vi "BlkReadFrame.vi"(0 "引用句柄输入":refnum<file>, 1 "datatype":i32, 2 "DST":T1, 3 "FrameWidth":i32, 4 "SkipFrame":i32, 5 "FrameHeight":i32) -> (6 "Image out":T1(plugin-control))   [LabVIEW 2011]
uses:
  <vilib>/vision/Image Controls.llb/IMAQ Image.ctl
panel:
  in  "数值 4":u8
  in  "数值 3":u32
  in  "数值 2":i16
  in  "数值":sgl
  in  "错误输入":errorcluster
  out "错误输出":errorcluster
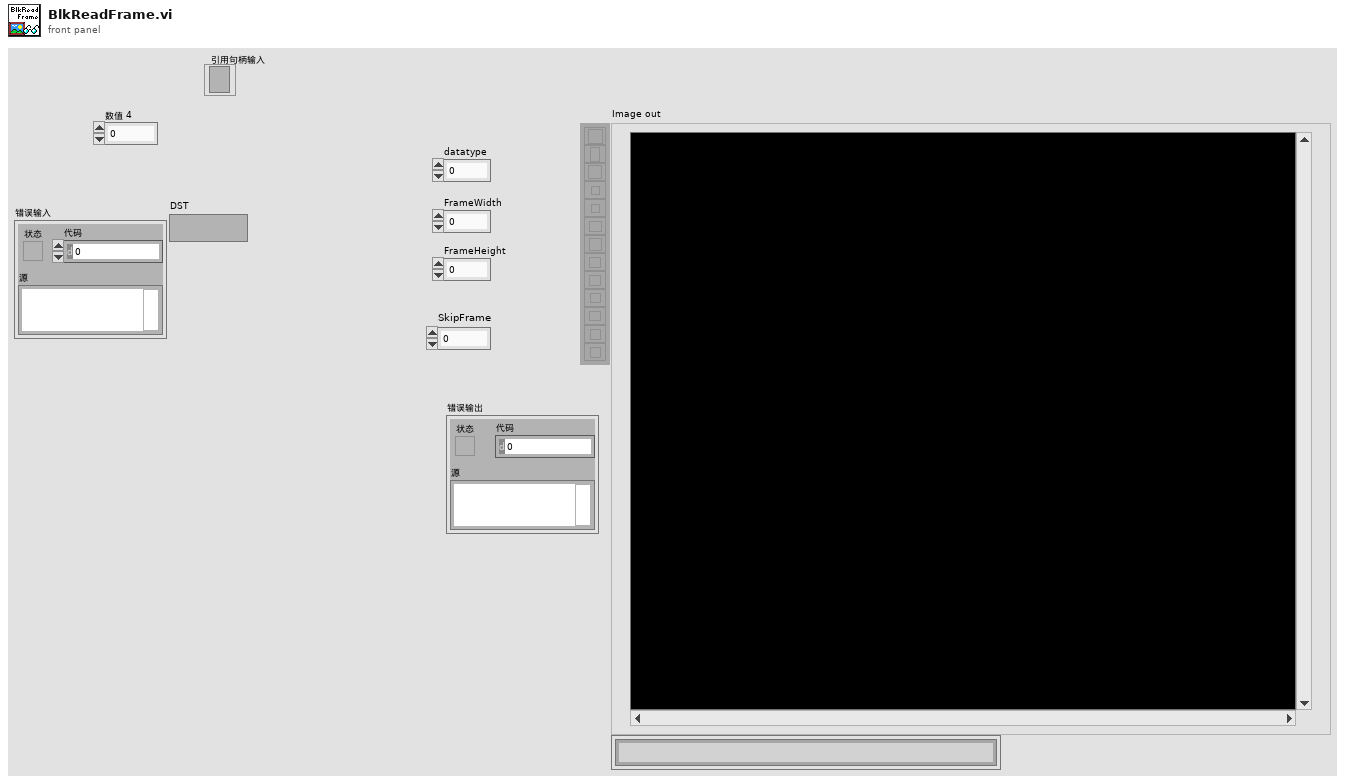
[diagram p1: front panel]
types:
  T1 = typedef "IMAQ Image.ctl" = refnum<image>
  T2 = enum16{"big-endian, network order", "native, host order", "little-endian"}
  T3 = typedef "Image Type" = u32
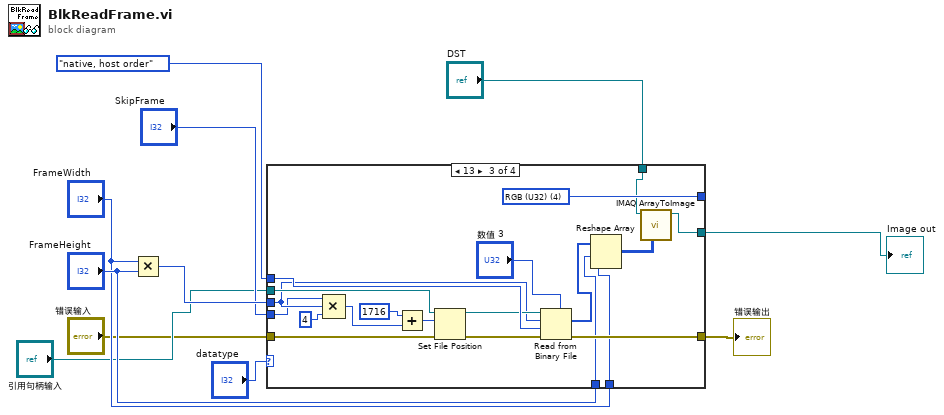
[diagram p0: block diagram]
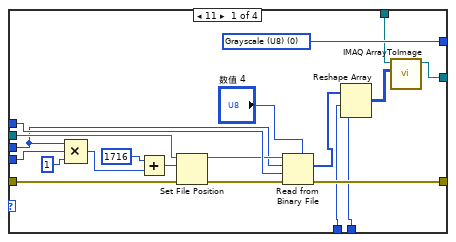
[diagram p2: hidden frame]
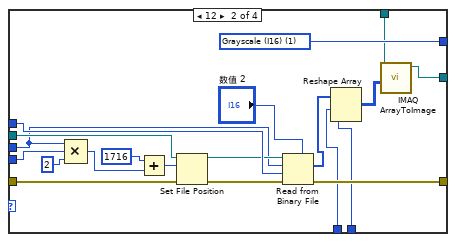
[diagram p3: hidden frame]
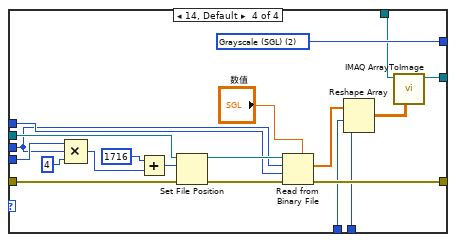
[diagram p4: hidden frame]
diagram:
  n1 = Multiply(x="FrameWidth", y="FrameHeight") -> (x*y=w8:i32)
  n2 = case shown="13" "datatype" {
    tunnel: [w31 w51 w71 w91] -> w11
    tunnel: T2."native, host order" ("字节顺序(0:big-endian, network order)") -> [w29 w49 w69 w80]
    tunnel: w8 -> [w18 w38 w61 w78]
    tunnel: [w28 w48 w68 w89] -> _
    tunnel: "错误输入" -> [w20 w40 w65 w82]
    tunnel: "引用句柄输入" -> [w21 w41 w64 w81]
    tunnel: "SkipFrame" -> [w19 w39 w58 w79]
    tunnel: "FrameHeight" -> [w15 w36 w55 w75]
    tunnel: "FrameWidth" -> [w14 w35 w54 w74]
    tunnel: "DST" -> [w12 w34 w53 w73]
    tunnel: [w17 w32 w52 w72] -> w3
    frame 11 {
      w28 = T3 0 items=["Grayscale (U8)", "Grayscale (I16)", "Grayscale (SGL)", "Complex (CSG)", "RGB (U32)", "HSL (U32)", "RGB (U64)", "Grayscale (U16)"] ("Image Type")
      n3 = Compound Arithmetic op=MULTIPLY(w18, w19, 1 ("y")) -> (w24:i32)
      n4 = Add(x=i64 1716 ("偏移量（字节）（0） 2"), y=w24) -> (x+y=w26:i64)
      n5 = Set File Position(offset (in bytes) (0)=w26, refnum=w21, error in=w20) -> (refnum out=w23:refnum<file>, error out=w22:errorcluster)  [unwired: 1 in]
      n6 = Read from Binary File(5:"数值 4", 8:w22, 9:w29, 10:w18, 11:w23) -> (0:w31:errorcluster, 2:w16:u8[])  [unwired: 1 in, 2 out]
      n7 = Reshape Array(w16, w15, w14) -> (w13:u8[][])
      n8 = call "IMAQ ArrayToImage"("Image Pixels (U8)"=w13, "Image"=w12) -> ("Image Out"=w17:T1)  [unwired: 8 in, 1 out]
    }
    frame 12 {
      w48 = T3 1 items=["Grayscale (U8)", "Grayscale (I16)", "Grayscale (SGL)", "Complex (CSG)", "RGB (U32)", "HSL (U32)", "RGB (U64)", "Grayscale (U16)"] ("Image Type")
      n9 = Compound Arithmetic op=MULTIPLY(w38, w39, 2 ("y")) -> (w44:i32)
      n10 = Add(x=i64 1716 ("偏移量（字节）（0） 2"), y=w44) -> (x+y=w46:i64)
      n11 = Set File Position(offset (in bytes) (0)=w46, refnum=w41, error in=w40) -> (refnum out=w43:refnum<file>, error out=w42:errorcluster)  [unwired: 1 in]
      n12 = Read from Binary File(5:"数值 2", 8:w42, 9:w49, 10:w38, 11:w43) -> (0:w51:errorcluster, 2:w37:i16[])  [unwired: 1 in, 2 out]
      n13 = Reshape Array(w37, w36, w35) -> (w33:i16[][])
      n14 = call "IMAQ ArrayToImage"("Image Pixels (I16)"=w33, "Image"=w34) -> ("Image Out"=w32:T1)  [unwired: 8 in, 1 out]
    }
    frame 13 {
      w68 = T3 4 items=["Grayscale (U8)", "Grayscale (I16)", "Grayscale (SGL)", "Complex (CSG)", "RGB (U32)", "HSL (U32)", "RGB (U64)", "Grayscale (U16)"] ("Image Type")
      n15 = Compound Arithmetic op=MULTIPLY(w58, w61, 4 ("y")) -> (w59:i32)
      n16 = Add(x=i64 1716 ("偏移量（字节）（0） 2"), y=w59) -> (x+y=w62:i64)
      n17 = Set File Position(offset (in bytes) (0)=w62, refnum=w64, error in=w65) -> (refnum out=w67:refnum<file>, error out=w66:errorcluster)  [unwired: 1 in]
      n18 = Read from Binary File(5:"数值 3", 8:w66, 9:w69, 10:w61, 11:w67) -> (0:w71:errorcluster, 2:w56:u32[])  [unwired: 1 in, 2 out]
      n19 = Reshape Array(w56, w55, w54) -> (w57:u32[][])
      n20 = call "IMAQ ArrayToImage"("Image Pixels (Float)"=w57, "Image"=w53) -> ("Image Out"=w52:T1)  [unwired: 8 in, 1 out]
    }
    frame 14, Default {
      w89 = T3 2 items=["Grayscale (U8)", "Grayscale (I16)", "Grayscale (SGL)", "Complex (CSG)", "RGB (U32)", "HSL (U32)", "RGB (U64)", "Grayscale (U16)"] ("Image Type")
      n21 = Compound Arithmetic op=MULTIPLY(w79, w78, 4 ("y")) -> (w85:i32)
      n22 = Add(x=i64 1716 ("偏移量（字节）（0） 2"), y=w85) -> (x+y=w87:i64)
      n23 = Set File Position(offset (in bytes) (0)=w87, refnum=w81, error in=w82) -> (refnum out=w84:refnum<file>, error out=w83:errorcluster)  [unwired: 1 in]
      n24 = Read from Binary File(5:"数值", 8:w83, 9:w80, 10:w78, 11:w84) -> (0:w91:errorcluster, 2:w77:sgl[])  [unwired: 1 in, 2 out]
      n25 = Reshape Array(w77, w75, w74) -> (w76:sgl[][])
      n26 = call "IMAQ ArrayToImage"("Image Pixels (Float)"=w76, "Image"=w73) -> ("Image Out"=w72:T1)  [unwired: 8 in, 1 out]
    }
  }
  "错误输出" <- w11
  "Image out" <- w3
